vi "String - XML String Decoding.vi"(11 "HEX String":string) -> (3 "XML String":string)   [LabVIEW 2013]
panel:
  # "E696 B0"
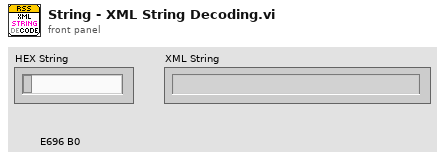
[diagram p1: front panel]
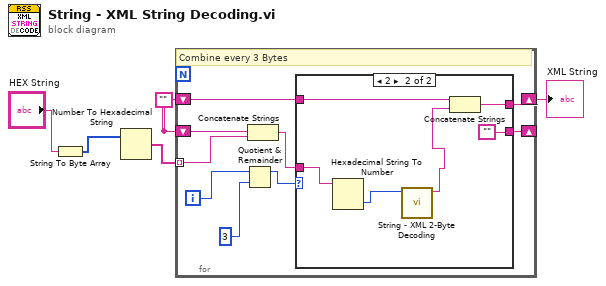
[diagram p0: block diagram]
diagram:
  w4 = ""
  n1 = String To Byte Array(string="HEX String") -> (unsigned byte array=w1:u8[])
  n2 = Number To Hexadecimal String(2:w1) -> (0:w2:string[])  [unwired: 1 in]
  n3 = for {
    shift-right: [w8] -> _
    shift-left: w4 -> [w13]
    tunnel: w2 -> [w14] mode=indexing
    shift-right: [w6] -> w5
    shift-left: w4 -> [w7]
    i -> [w12]
    # "Combine every 3 Bytes"
    n4 = Quotient & Remainder(x=w12, y=3) -> (x-y*floor(x/y)=w10:i32)  [unwired: 1 out]
    n5 = Concatenate Strings(w13, w14) -> (w9:string)
    n6 = case shown="2" w10 {
      tunnel: w9 -> [w16 w19]
      tunnel: [w16 ""] -> w8
      tunnel: w7 -> [w15 w21]
      tunnel: [w15 w20] -> w6
      frame 0, Default {
      }
      frame 2 {
        n7 = Hexadecimal String To Number(string=w19) -> (number=w18:u32)  [unwired: 2 in, 1 out]
        n8 = call "String - XML 2-Byte Decoding.vi"("Number In (3-Bytes -24bits)"=w18) -> ("Output (\\ Format)"=w17:string)  [unwired: 7 in, 2 out]
        n9 = Concatenate Strings(w21, w17) -> (w20:string)
      }
    }
  }
  "XML String" <- w5
